vi "Get Current Message Text Format.vi"(7 "Error In":errorcluster, 9 "Text Format":T1) -> (0 "Error Out":errorcluster, 2 "Message Formatting":T2={"Font"="", "Text Color"=enum."Unchanged", "Background Color"=enum."Unchanged", "Style"=enum."Regular", "Font Size"=6.0, "Alignment"=enum."Left"} {"Font Size" min=6.0 step=1.0})   [LabVIEW 2021, in "Notebook.lvlib"]
uses:
  Notebook.lvlib
  Rich Text Box/Text Formatting.ctl
  Rich Text Box/Text Colors.ctl
  Rich Text Box/Text Style.ctl
  Rich Text Box/Text Alignment.ctl
  Rich Text Box/Text Format List.ctl
  Notebook Parameters List.ctl
  Variant/Variant to Data/Variant to String.vi
  Variant/Variant to Data/Variant to Data.lvlib
  Rich Text Box/Rich Text Box.lvlib
panel:
  # "see the License on the block diagram (Ctrl+E or Window:Show Block Diagram)"
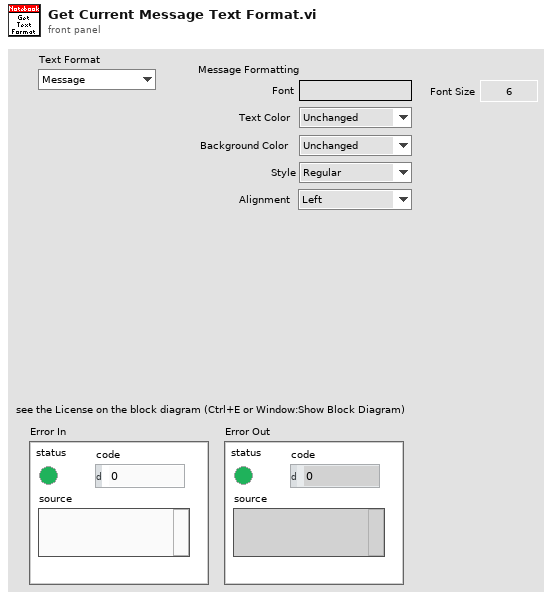
[diagram p1: front panel]
types:
  T1 = typedef "Notebook.lvlib/Text Format List.ctl" = enum16{"Message", "Result", "Error", "Setting", "Verbose", "Warning"}
  T2 = typedef "Rich Text Box.lvlib/Text Formatting.ctl" = cluster{"Font":string, "Text Color":T3, "Background Color":T3, "Style":T4, "Font Size":dbl, "Alignment":T5}
  T3 = typedef "Rich Text Box.lvlib/Text Colors.ctl" = enum16{"Unchanged", "Black", "Blue", "Cyan", "Maroon", "Gray", "Violet", "Green", "Light Green", "Orange", "Yellow", "Magenta", "Red", "White"}
  T4 = typedef "Rich Text Box.lvlib/Text Style.ctl" = enum16{"Regular", "Bold", "Italic", "Underline", "Strikeout"}
  T5 = typedef "Rich Text Box.lvlib/Text Alignment.ctl" = enum16{"Left", "Right", "Center"}
  T6 = typedef "Notebook.lvlib/Notebook Parameters List.ctl" = enum16{"First Opening?", "Saved Notebook?", "Saved Notebook Path", "Beep on Error?", "Notebook Themes", "Current Theme Name"}
  T7 = typedef "Notebook.lvlib/Notebook Theme.ctl" = cluster{"Theme Name":string, "[Named Text Styles]":T8[], "Page Color":T3}
  T8 = typedef "Notebook.lvlib/Named Text Style.ctl" = cluster{"Text Formatting":T2, "Text Style Name":string}
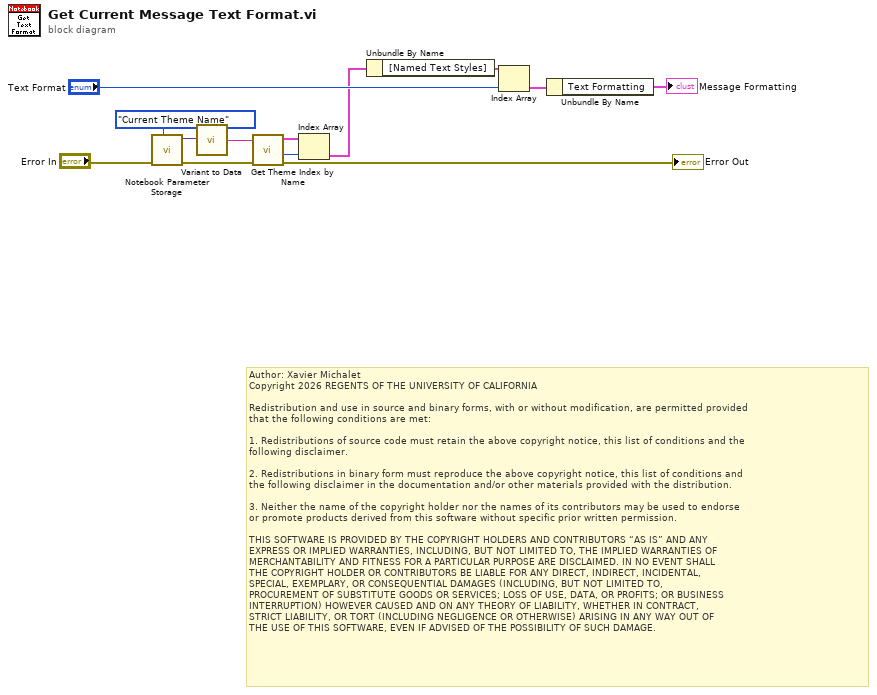
[diagram p0: block diagram]
diagram:
  # "Author: Xavier Michalet\nCopyright 2026 REGENTS OF THE UNIVERSITY OF CALIFORNIA\n\nRedistribution and use in source and binary forms, with or without modification, are permitted provided\nthat the following conditions are met:\n\n1. Redistributions of source code must retain the above copyright notice, this list of conditions and the\nfollowing disclaimer.\n\n2. Redistributions in binary form must reproduce the above copyright notice, this list of conditions and\nthe following disclaimer in the documentation and/or other materials provided with the distribution.\n\n3. Neither the name of the copyright holder nor the names of its contributors may be used to endorse \nor promote products derived from this software without specific prior written permission.\n\nTHIS SOFTWARE IS PROVIDED BY THE COPYRIGHT HOLDERS AND CONTRIBUTORS “AS IS” AND ANY \nEXPRESS OR IMPLIED WARRANTIES, INCLUDING, BUT NOT LIMITED TO, THE IMPLIED WARRANTIES OF\nMERCHANTABILITY AND FITNESS FOR A PARTICULAR PURPOSE ARE DISCLAIMED. IN NO EVENT SHALL\nTHE COPYRIGHT HOLDER OR CONTRIBUTORS BE LIABLE FOR ANY DIRECT, INDIRECT, INCIDENTAL, \nSPECIAL, EXEMPLARY, OR CONSEQUENTIAL DAMAGES (INCLUDING, BUT NOT LIMITED TO, \nPROCUREMENT OF SUBSTITUTE GOODS OR SERVICES; LOSS OF USE, DATA, OR PROFITS; OR BUSINESS\nINTERRUPTION) HOWEVER CAUSED AND ON ANY THEORY OF LIABILITY, WHETHER IN CONTRACT, \nSTRICT LIABILITY, OR TORT (INCLUDING NEGLIGENCE OR OTHERWISE) ARISING IN ANY WAY OUT OF\nTHE USE OF THIS SOFTWARE, EVEN IF ADVISED OF THE POSSIBILITY OF SUCH DAMAGE."
  n1 = call "Notebook Parameter Storage.vi"("Notebook Parameter List"=Notebook_Parameters_List."Current Theme Name", "Error In"="Error In") -> ("Error Out"=w8:errorcluster, "Data out"=w6:variant)  [unwired: 8 in]
  n2 = call-poly "Variant to Data.vi"("Variant"=w6) -> ("String"=w5:string)  [unwired: 8 in]
  n3 = call "Get Theme Index by Name.vi"("error in (no error)"=w8, "Theme Name"=w5) -> ("error out"=→"Error Out":errorcluster, "Theme Index"=w3:i32, "Theme Array"=w4:T7[])  [unwired: 6 in, 1 out]
  n4 = Index Array(array=w4, index=w3) -> (element=w2:T7)
  n5 = Unbundle By Name(w2) -> ("[Named Text Styles]"=w12:T8[])
  n6 = Index Array(array=w12, index="Text Format") -> (element=w11:T8)
  n7 = Unbundle By Name(w11) -> ("Text Formatting"=→"Message Formatting":T2)
